vi "CallingVI.vi"() -> ()   [LabVIEW 2012]
uses:
  TimerCommands.ctl
panel:
  in  "目标时间(s)":dbl
  out "已用时间":dbl
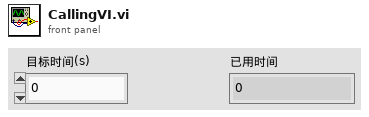
[diagram p1: front panel]
types:
  T1 = typedef "TimerCommands.ctl" = enum16{"开始", "检查时间"}
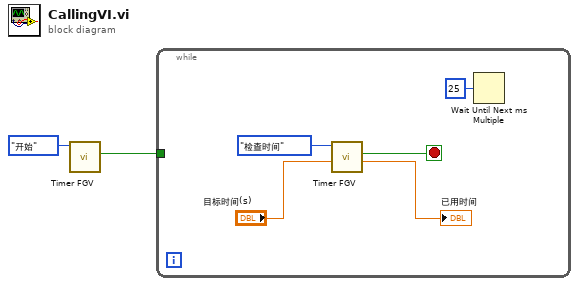
[diagram p0: block diagram]
diagram:
  n1 = call "Timer FGV.vi"("定时器命令"=TimerCommands."开始") -> ("完成？"=w2:bool)  [unwired: 9 in, 1 out]
  n2 = while {
    tunnel: w2 -> [_]
    stop <- w6 stop-if-true
    n3 = call "Timer FGV.vi"("目标时间(s)"="目标时间(s)", "定时器命令"=TimerCommands."检查时间") -> ("已用时间"=→"已用时间":dbl, "完成？"=w6:bool)  [unwired: 8 in]
    n4 = Wait Until Next ms Multiple ("等待下一个整数倍毫秒")(millisecond multiple=u32 25 ("毫秒倍数")) -> ()  [unwired: 1 out]
  }
